vi "TWT spec. file I_O.vi"(8 "error in":errorcluster, 10 "TWT type":string, 11 "Enum":T2(ring)=enum."read TWT spec.") -> (0 "error out":errorcluster, 2 "TWT spec":T1, 3 "TWT types":string[](array[string]))   [LabVIEW 2014]
uses:
  Controls/TWT spec..ctl
  <vilib>/Utility/config.llb/Read Key (String).vi
  <vilib>/Utility/config.llb/NI_LVConfig.lvlib
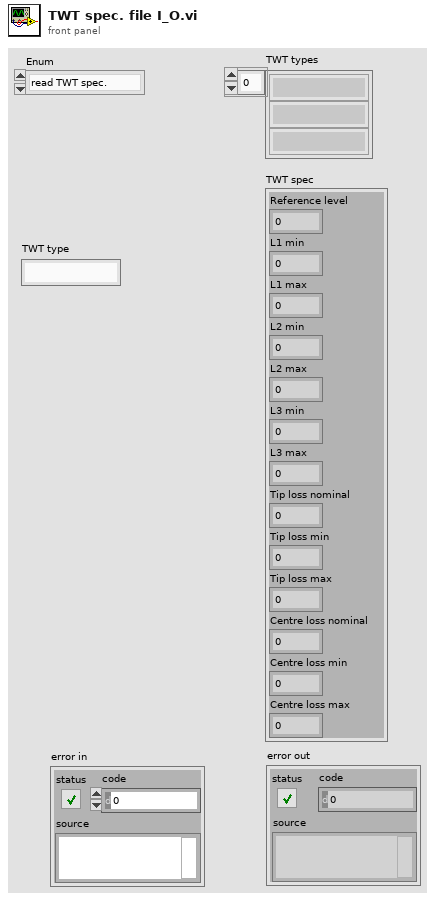
[diagram p1: front panel]
types:
  T1 = typedef "TWT spec..ctl" = cluster{"Reference level":dbl, "L1 min":dbl, "L1 max":dbl, "L2 min":dbl, "L2 max":dbl, "L3 min":dbl, "L3 max":dbl, "Tip loss nominal":dbl, "Tip loss min":dbl, "Tip loss max":dbl, "Centre loss nominal":dbl, "Centre loss min":dbl, "Centre loss max":dbl}
  T2 = enum16{"get TWT types", "read TWT spec.", "save TWT spec.", "remove TWT spec."}
  T3 = typedef "NI_LVConfig.lvlib/Config Data RefNum.ctl" = refnum<k1>
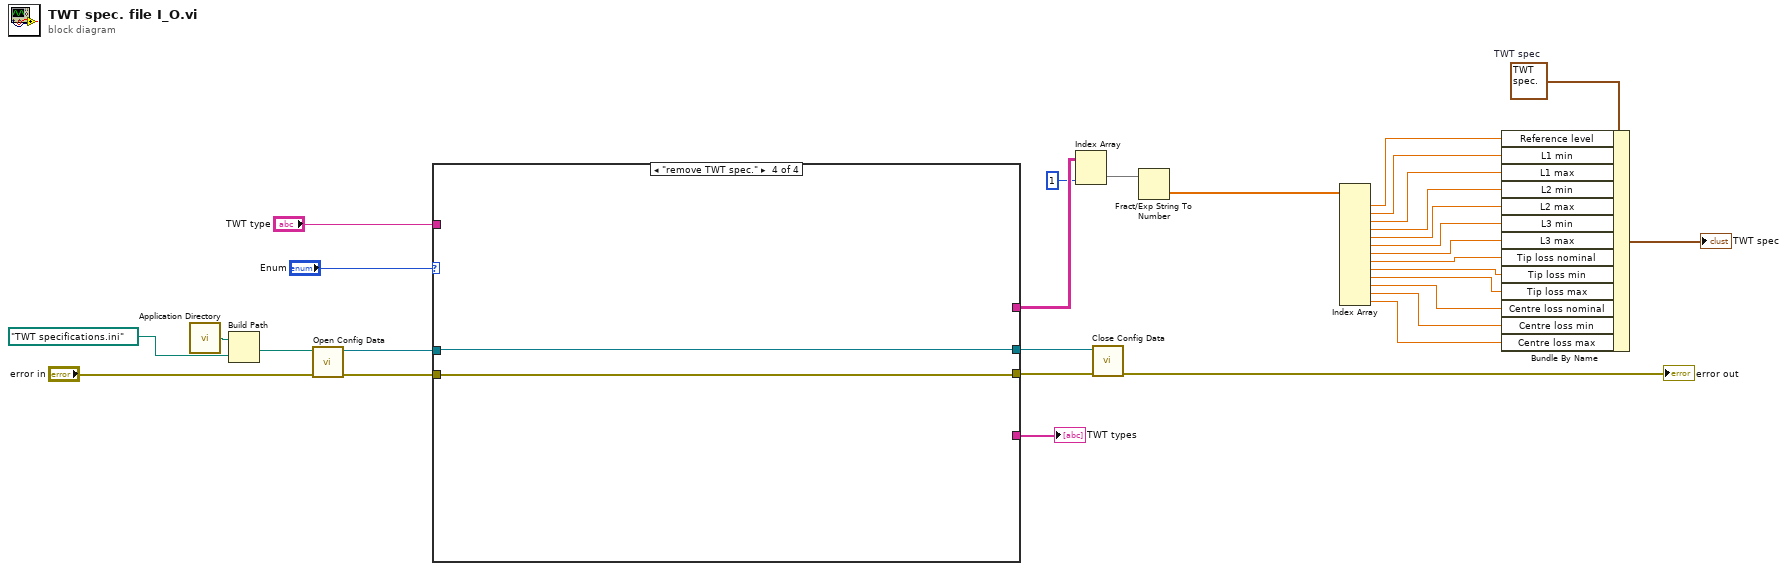
[diagram p0: block diagram]
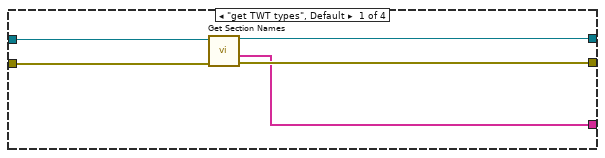
[diagram p2: hidden frame]
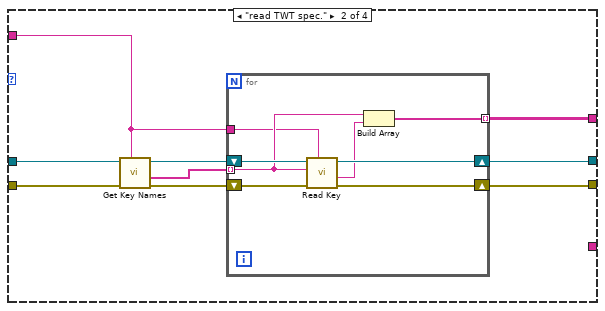
[diagram p3: hidden frame]
diagram:
  w1 = T1 {"Reference level"=0.0, "L1 min"=0.0, "L1 max"=0.0, "L2 min"=0.0, "L2 max"=0.0, "L3 min"=0.0, "L3 max"=0.0, "Tip loss nominal"=0.0, "Tip loss min"=0.0, "Tip loss max"=0.0, "Centre loss nominal"=0.0, "Centre loss min"=0.0, "Centre loss max"=0.0}  # TWT spec
  n1 = call <vilib>:"Application Directory.vi"() -> ("Application Directory"=w31:path)
  n2 = Build Path(base path=w31, name or relative path=path "TWT specifications.ini") -> (appended path=w26:path)
  n3 = call <vilib>:"Open Config Data.vi"("error in (no error)"="error in", "configuration file path"=w26) -> ("error out"=w24:errorcluster, "refnum"=w25:T3)  [unwired: 7 in, 1 out]
  n4 = case shown="\"remove TWT spec.\"" "Enum" {
    tunnel: w25 -> [w34 w44 w55 w56]
    tunnel: [w36 w41 w55 w56] -> w29
    tunnel: [w35 w40 w54 w57] -> w28
    tunnel: w24 -> [w33 w45 w54 w57]
    tunnel: "TWT type" -> [_ w38 _ _]
    tunnel: [_ w37 _ _] -> w21
    tunnel: [w32 _ _ _] -> w22
    frame "get TWT types", Default {
      n5 = call <vilib>:"Get Section Names.vi"("error in (no error)"=w33, "refnum"=w34) -> ("error out"=w35:errorcluster, "section names"=w32:string[], "refnum out"=w36:T3)  [unwired: 7 in]
    }
    frame "read TWT spec." {
      n6 = call <vilib>:"Get Key Names.vi"("section"=w38, "error in (no error)"=w45, "refnum"=w44) -> ("error out"=w39:errorcluster, "key names"=w43:string[], "refnum out"=w42:T3)  [unwired: 5 in, 1 out]
      n7 = for {
        tunnel: w43 -> [w49] mode=indexing
        shift-right: [w52] -> w41
        shift-left: w42 -> [w53]
        shift-right: [w51] -> w40
        shift-left: w39 -> [w50]
        tunnel: [w47] -> w37 mode=indexing
        tunnel: w38 -> [w46]
        n8 = call-poly <vilib>:"Read Key.vi"("section"=w46, "error in (no error)"=w50, "key"=w49, "refnum"=w53) -> ("error out"=w51:errorcluster, "value"=w48:string, "refnum out"=w52:T3)  [unwired: 4 in, 1 out]
        n9 = Build Array(w49, w48) -> (w47:string[])
      }
    }
    frame "save TWT spec." {
    }
    frame "remove TWT spec." {
    }
  }
  "TWT types" <- w22
  n10 = Index Array(array=w21, index (col)=1 ("disabled index (col)")) -> (element=w19:string[])  [unwired: 1 in]
  n11 = call <vilib>:"Close Config Data.vi"("error in (no error)"=w28, "refnum"=w29) -> ("error out"=→"error out":errorcluster)  [unwired: 8 in, 1 out]
  n12 = Fract/Exp String To Number(string=w19) -> (number=w18:dbl[])  [unwired: 3 in, 1 out]
  n13 = Index Array(array=w18) -> (element #1=w17:dbl, element #2=w16:dbl, element #3=w15:dbl, element #4=w14:dbl, element #5=w13:dbl, element #6=w12:dbl, element #7=w11:dbl, element #8=w10:dbl, element #9=w9:dbl, element #10=w8:dbl, element #11=w7:dbl, element #12=w6:dbl, element #13=w5:dbl)  [unwired: 13 in]
  n14 = Bundle By Name(cluster=w1, "Reference level"=w17, "L1 min"=w16, "L1 max"=w15, "L2 min"=w14, "L2 max"=w13, "L3 min"=w12, "L3 max"=w11, "Tip loss nominal"=w10, "Tip loss min"=w9, "Tip loss max"=w8, "Centre loss nominal"=w7, "Centre loss min"=w6, "Centre loss max"=w5) -> (→"TWT spec":T1)
